vi "Create Pattern Script(Special Frames).vi"(7 "Special Frame Type":T1, 8 "error in (no error)":errorcluster, 10 "Num of Timeset":u32, 11 "SPI Root Pattern Creator in":refnum<class "SPI Root Pattern Creator.lvclass">) -> (0 "error out":errorcluster, 2 "String out":string, 3 "SPI Root Pattern Creator out":refnum<class "SPI Root Pattern Creator.lvclass">)   [LabVIEW 2018, in "SPI Root Pattern Creator.lvlib" / "SPI Root Pattern Creator.lvclass"]
uses:
  SPI Root Pattern Creator.lvclass
  Special Frame Type.ctl
  Interfaces/Protocol Interface.lvlibp/Interfaces/Protocol Interface/Pin State.ctl
  Interfaces/Protocol Interface.lvlibp/Interfaces/Protocol Interface/Protocol Interface.lvclass
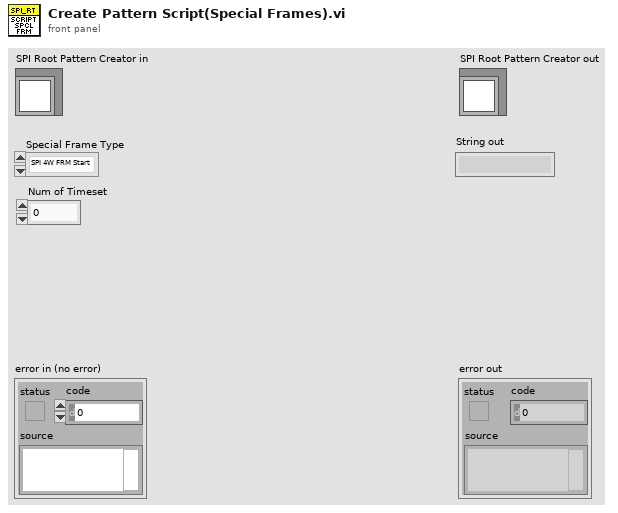
[diagram p1: front panel]
types:
  T1 = typedef "SPI Root Pattern Creator.lvlib/SPI Root Pattern Creator.lvclass/Special Frame Type.ctl" = enum16{"SPI 4W FRM Start", "SPI 4W Wait", "SPI 4W FRM End", "SPI 4W Write Cmd", "SPI Rd Collect Cmd", "SPI Rd Value Cmd", "SPI 3W FRM Start", "SPI 3W Write Cmd", "SPI 3W FRM End", "SPI 3W Wait", "SPI 3W Rd Cmd"}
  T2 = typedef "Protocol Interface.lvlibp/Protocol Interface.lvclass/Pin State.ctl" = enum16{"0", "1", "L", "H", "X", "V", "D", "M"}
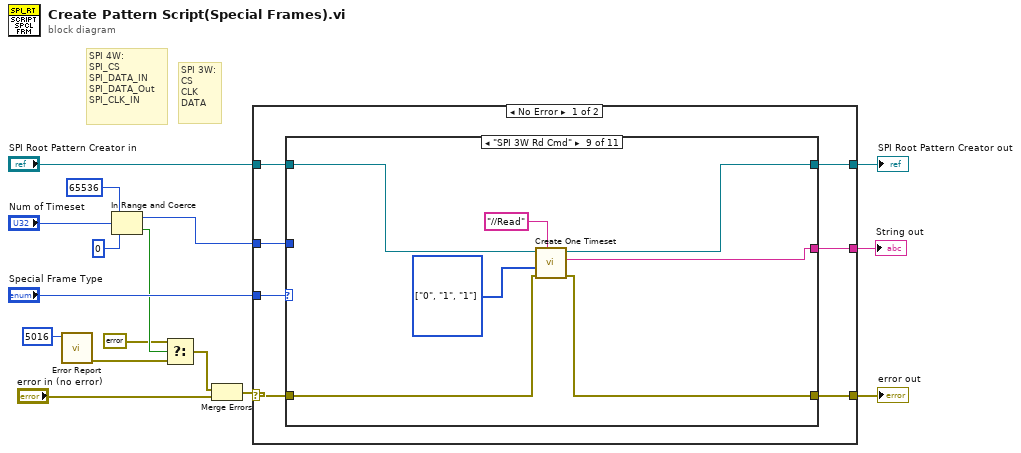
[diagram p0: block diagram]
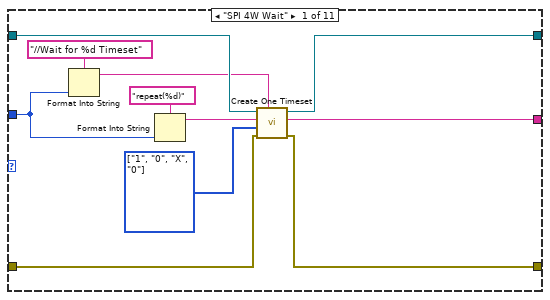
[diagram p2: hidden frame]
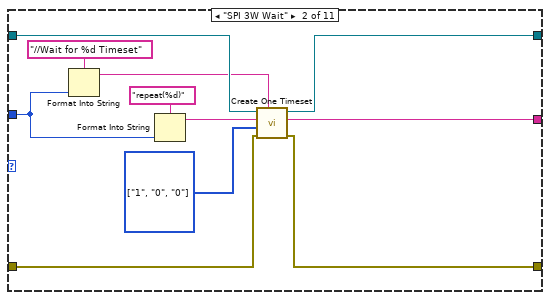
[diagram p3: hidden frame]
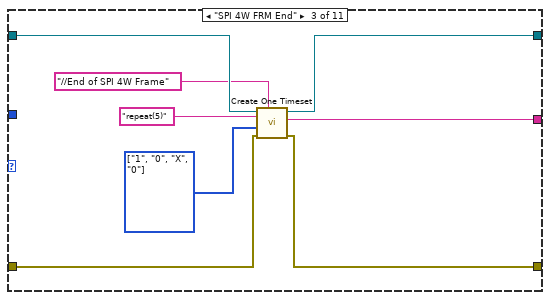
[diagram p4: hidden frame]
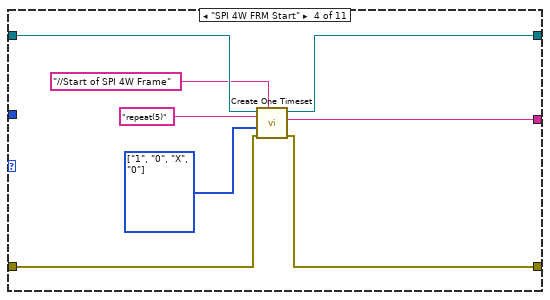
[diagram p5: hidden frame]
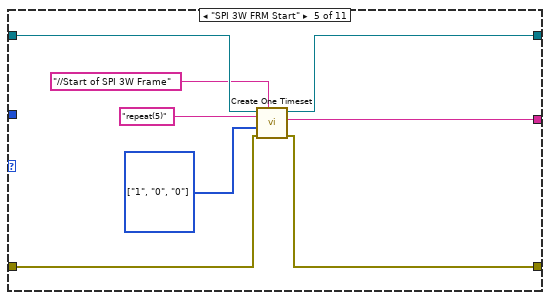
[diagram p6: hidden frame]
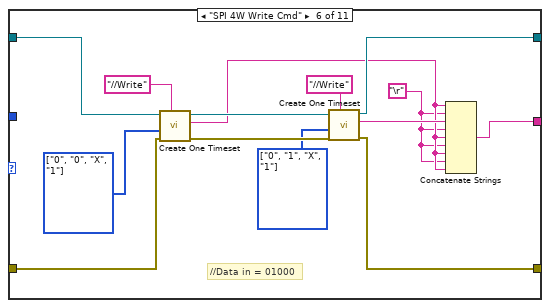
[diagram p7: hidden frame]
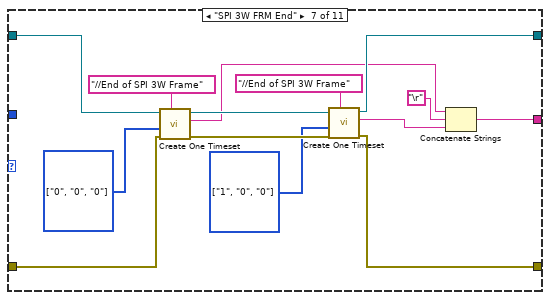
[diagram p8: hidden frame]
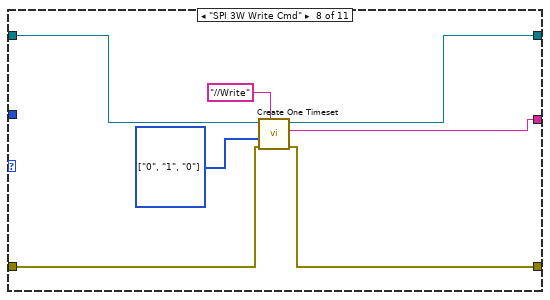
[diagram p9: hidden frame]
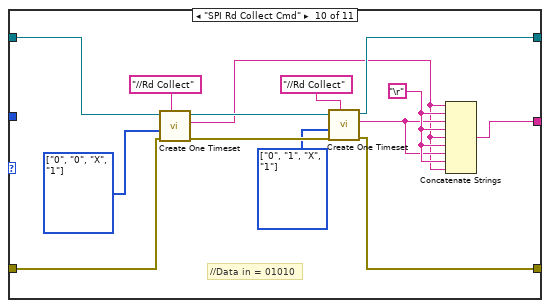
[diagram p10: hidden frame]
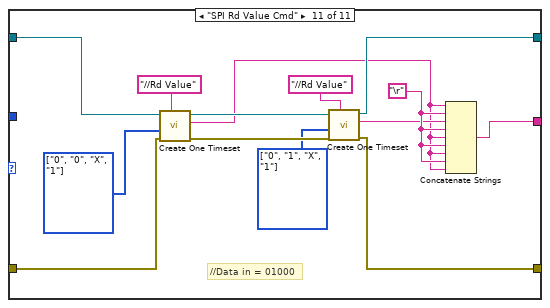
[diagram p11: hidden frame]
diagram:
  # "SPI 3W:\nCS\nCLK\nDATA"
  # "SPI 4W:\nSPI_CS\nSPI_DATA_IN\nSPI_DATA_Out\nSPI_CLK_IN"
  n1 = call "Error Report.vi"("Error Code"=i16 5016) -> ("error out"=w8:errorcluster)  [unwired: 10 in]
  n2 = In Range and Coerce(upper limit=u32 65536, x="Num of Timeset", lower limit=u32 0 ("upper limit")) -> (coerced(x)=w6:u32, In Range?=w7:bool)
  n3 = Select(t=errorcluster {"status"=FALSE, "code"=0, "source"=""}, s=w7, f=w8) -> (s? t:f=w3:errorcluster)
  n4 = Merge Errors(w3, "error in (no error)") -> (w2:errorcluster)
  n5 = case shown="No Error" w2 {
    selector: w2 -> [w20 w141]
    tunnel: [w17 w141] -> w16
    tunnel: [w19 w140] -> w14
    tunnel: "SPI Root Pattern Creator in" -> [w22 w140]
    tunnel: "Special Frame Type" -> [w23 _]
    tunnel: w6 -> [w21 _]
    tunnel: [w18 _] -> w1
    frame No Error {
      n6 = case shown="\"SPI 3W Rd Cmd\"" w23 {
        tunnel: w22 -> [w30 w41 w53 w61 w69 w81 w95 w102 w109 w123 w137]
        tunnel: w21 -> [w32 w43 _ _ _ _ _ _ _ _ _]
        tunnel: w20 -> [w27 w38 w51 w59 w67 w79 w93 w104 w111 w121 w135]
        tunnel: [w26 w37 w50 w58 w66 w83 w97 w101 w108 w125 w139] -> w19
        tunnel: [w25 w36 w49 w57 w65 w70 w88 w98 w105 w115 w129] -> w18
        tunnel: [w24 w35 w48 w56 w64 w82 w96 w103 w110 w124 w138] -> w17
        frame "SPI 4W Wait" {
          w28 = T2[] [enum."1", enum."0", enum."X", enum."0"] items=["0", "1", "L", "H", "X", "V", "D", "M"] ("PinStates")
          n7 = Format Into String(format string="//Wait for %d Timeset", w32) -> (resulting string=w29:string)  [unwired: 2 in, 1 out]
          n8 = Format Into String(format string="repeat(%d)", w32) -> (resulting string=w31:string)  [unwired: 2 in, 1 out]
          n9 = call-dynamic "Create One Timeset.vi"("Notes"=w29, "error in (no error)"=w27, "PinStates"=w28, "OpCode"=w31, "SPI Root Pattern Creator in"=w30) -> ("error out"=w24:errorcluster, "String  out"=w25:string, "SPI Root Pattern Creator out"=w26:refnum<class "SPI Root Pattern Creator.lvclass">)  [unwired: 4 in]
        }
        frame "SPI 3W Wait" {
          w39 = T2[] [enum."1", enum."0", enum."0"] items=["0", "1", "L", "H", "X", "V", "D", "M"] ("PinStates")
          n10 = Format Into String(format string="//Wait for %d Timeset", w43) -> (resulting string=w40:string)  [unwired: 2 in, 1 out]
          n11 = Format Into String(format string="repeat(%d)", w43) -> (resulting string=w42:string)  [unwired: 2 in, 1 out]
          n12 = call-dynamic "Create One Timeset.vi"("Notes"=w40, "error in (no error)"=w38, "PinStates"=w39, "OpCode"=w42, "SPI Root Pattern Creator in"=w41) -> ("error out"=w35:errorcluster, "String  out"=w36:string, "SPI Root Pattern Creator out"=w37:refnum<class "SPI Root Pattern Creator.lvclass">)  [unwired: 4 in]
        }
        frame "SPI 4W FRM End" {
          w52 = T2[] [enum."1", enum."0", enum."X", enum."0"] items=["0", "1", "L", "H", "X", "V", "D", "M"] ("PinStates")
          n13 = call-dynamic "Create One Timeset.vi"("Notes"="//End of SPI 4W Frame" ("format string"), "error in (no error)"=w51, "PinStates"=w52, "OpCode"="repeat(5)" ("format string"), "SPI Root Pattern Creator in"=w53) -> ("error out"=w48:errorcluster, "String  out"=w49:string, "SPI Root Pattern Creator out"=w50:refnum<class "SPI Root Pattern Creator.lvclass">)  [unwired: 4 in]
        }
        frame "SPI 4W FRM Start" {
          w60 = T2[] [enum."1", enum."0", enum."X", enum."0"] items=["0", "1", "L", "H", "X", "V", "D", "M"] ("PinStates")
          n14 = call-dynamic "Create One Timeset.vi"("Notes"="//Start of SPI 4W Frame" ("format string"), "error in (no error)"=w59, "PinStates"=w60, "OpCode"="repeat(5)" ("format string"), "SPI Root Pattern Creator in"=w61) -> ("error out"=w56:errorcluster, "String  out"=w57:string, "SPI Root Pattern Creator out"=w58:refnum<class "SPI Root Pattern Creator.lvclass">)  [unwired: 4 in]
        }
        frame "SPI 3W FRM Start" {
          w68 = T2[] [enum."1", enum."0", enum."0"] items=["0", "1", "L", "H", "X", "V", "D", "M"] ("PinStates")
          n15 = call-dynamic "Create One Timeset.vi"("Notes"="//Start of SPI 3W Frame" ("format string"), "error in (no error)"=w67, "PinStates"=w68, "OpCode"="repeat(5)" ("format string"), "SPI Root Pattern Creator in"=w69) -> ("error out"=w64:errorcluster, "String  out"=w65:string, "SPI Root Pattern Creator out"=w66:refnum<class "SPI Root Pattern Creator.lvclass">)  [unwired: 4 in]
        }
        frame "SPI 4W Write Cmd" {
          w71 = "\r"
          w74 = T2[] [enum."0", enum."1", enum."X", enum."1"] items=["0", "1", "L", "H", "X", "V", "D", "M"] ("PinStates")
          w76 = T2[] [enum."0", enum."0", enum."X", enum."1"] items=["0", "1", "L", "H", "X", "V", "D", "M"] ("PinStates")
          # "//Data in = 01000"
          n16 = call-dynamic "Create One Timeset.vi"("Notes"="//Write", "error in (no error)"=w79, "PinStates"=w76, "SPI Root Pattern Creator in"=w81) -> ("error out"=w78:errorcluster, "String  out"=w72:string, "SPI Root Pattern Creator out"=w80:refnum<class "SPI Root Pattern Creator.lvclass">)  [unwired: 5 in]
          n17 = call-dynamic "Create One Timeset.vi"("Notes"="//Write", "error in (no error)"=w78, "PinStates"=w74, "SPI Root Pattern Creator in"=w80) -> ("error out"=w82:errorcluster, "String  out"=w73:string, "SPI Root Pattern Creator out"=w83:refnum<class "SPI Root Pattern Creator.lvclass">)  [unwired: 5 in]
          n18 = Concatenate Strings(w72, w71, w73, w71, w72, w71, w72, w71, w72) -> (w70:string)
        }
        frame "SPI 3W FRM End" {
          w87 = T2[] [enum."1", enum."0", enum."0"] items=["0", "1", "L", "H", "X", "V", "D", "M"] ("PinStates")
          w90 = T2[] [enum."0", enum."0", enum."0"] items=["0", "1", "L", "H", "X", "V", "D", "M"] ("PinStates")
          n19 = call-dynamic "Create One Timeset.vi"("Notes"="//End of SPI 3W Frame", "error in (no error)"=w93, "PinStates"=w90, "SPI Root Pattern Creator in"=w95) -> ("error out"=w92:errorcluster, "String  out"=w86:string, "SPI Root Pattern Creator out"=w94:refnum<class "SPI Root Pattern Creator.lvclass">)  [unwired: 5 in]
          n20 = call-dynamic "Create One Timeset.vi"("Notes"="//End of SPI 3W Frame", "error in (no error)"=w92, "PinStates"=w87, "SPI Root Pattern Creator in"=w94) -> ("error out"=w96:errorcluster, "String  out"=w84:string, "SPI Root Pattern Creator out"=w97:refnum<class "SPI Root Pattern Creator.lvclass">)  [unwired: 5 in]
          n21 = Concatenate Strings(w86, "\r", w84) -> (w88:string)
        }
        frame "SPI 3W Write Cmd" {
          w99 = T2[] [enum."0", enum."1", enum."0"] items=["0", "1", "L", "H", "X", "V", "D", "M"] ("PinStates")
          n22 = call-dynamic "Create One Timeset.vi"("Notes"="//Write", "error in (no error)"=w104, "PinStates"=w99, "SPI Root Pattern Creator in"=w102) -> ("error out"=w103:errorcluster, "String  out"=w98:string, "SPI Root Pattern Creator out"=w101:refnum<class "SPI Root Pattern Creator.lvclass">)  [unwired: 5 in]
        }
        frame "SPI 3W Rd Cmd" {
          w106 = T2[] [enum."0", enum."1", enum."1"] items=["0", "1", "L", "H", "X", "V", "D", "M"] ("PinStates")
          n23 = call-dynamic "Create One Timeset.vi"("Notes"="//Read", "error in (no error)"=w111, "PinStates"=w106, "SPI Root Pattern Creator in"=w109) -> ("error out"=w110:errorcluster, "String  out"=w105:string, "SPI Root Pattern Creator out"=w108:refnum<class "SPI Root Pattern Creator.lvclass">)  [unwired: 5 in]
        }
        frame "SPI Rd Collect Cmd" {
          w114 = "\r"
          w116 = T2[] [enum."0", enum."1", enum."X", enum."1"] items=["0", "1", "L", "H", "X", "V", "D", "M"] ("PinStates")
          w118 = T2[] [enum."0", enum."0", enum."X", enum."1"] items=["0", "1", "L", "H", "X", "V", "D", "M"] ("PinStates")
          # "//Data in = 01010"
          n24 = call-dynamic "Create One Timeset.vi"("Notes"="//Rd Collect", "error in (no error)"=w121, "PinStates"=w118, "SPI Root Pattern Creator in"=w123) -> ("error out"=w120:errorcluster, "String  out"=w112:string, "SPI Root Pattern Creator out"=w122:refnum<class "SPI Root Pattern Creator.lvclass">)  [unwired: 5 in]
          n25 = call-dynamic "Create One Timeset.vi"("Notes"="//Rd Collect", "error in (no error)"=w120, "PinStates"=w116, "SPI Root Pattern Creator in"=w122) -> ("error out"=w124:errorcluster, "String  out"=w113:string, "SPI Root Pattern Creator out"=w125:refnum<class "SPI Root Pattern Creator.lvclass">)  [unwired: 5 in]
          n26 = Concatenate Strings(w112, w114, w113, w114, w112, w114, w113, w114, w112) -> (w115:string)
        }
        frame "SPI Rd Value Cmd" {
          w128 = "\r"
          w130 = T2[] [enum."0", enum."1", enum."X", enum."1"] items=["0", "1", "L", "H", "X", "V", "D", "M"] ("PinStates")
          w132 = T2[] [enum."0", enum."0", enum."X", enum."1"] items=["0", "1", "L", "H", "X", "V", "D", "M"] ("PinStates")
          # "//Data in = 01000"
          n27 = call-dynamic "Create One Timeset.vi"("Notes"="//Rd Value", "error in (no error)"=w135, "PinStates"=w132, "SPI Root Pattern Creator in"=w137) -> ("error out"=w134:errorcluster, "String  out"=w126:string, "SPI Root Pattern Creator out"=w136:refnum<class "SPI Root Pattern Creator.lvclass">)  [unwired: 5 in]
          n28 = call-dynamic "Create One Timeset.vi"("Notes"="//Rd Value", "error in (no error)"=w134, "PinStates"=w130, "SPI Root Pattern Creator in"=w136) -> ("error out"=w138:errorcluster, "String  out"=w127:string, "SPI Root Pattern Creator out"=w139:refnum<class "SPI Root Pattern Creator.lvclass">)  [unwired: 5 in]
          n29 = Concatenate Strings(w126, w128, w127, w128, w126, w128, w126, w128, w126) -> (w129:string)
        }
      }
    }
    frame Error {
    }
  }
  "error out" <- w16
  "SPI Root Pattern Creator out" <- w14
  "String out" <- w1
